vi "Get Column Config.vi"(8 "error in (no error)":errorcluster, 11 "Column Parent in":refnum<class "Column Parent.lvclass">) -> (0 "error out":errorcluster, 2 "Column Configuration":refnum<class "Column Configuration.lvclass">, 3 "Column Parent out":refnum<class "Column Parent.lvclass">)   [LabVIEW 2020, in "Basic Columns.lvlib" / "Column Parent.lvclass"]
uses:
  Column Parent.lvclass
  Column Interface/Column Configuration Interface Class/Column Configuration.lvclass
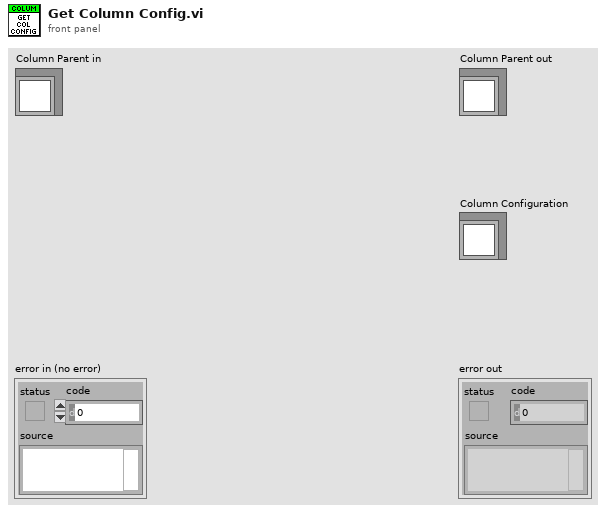
[diagram p1: front panel]
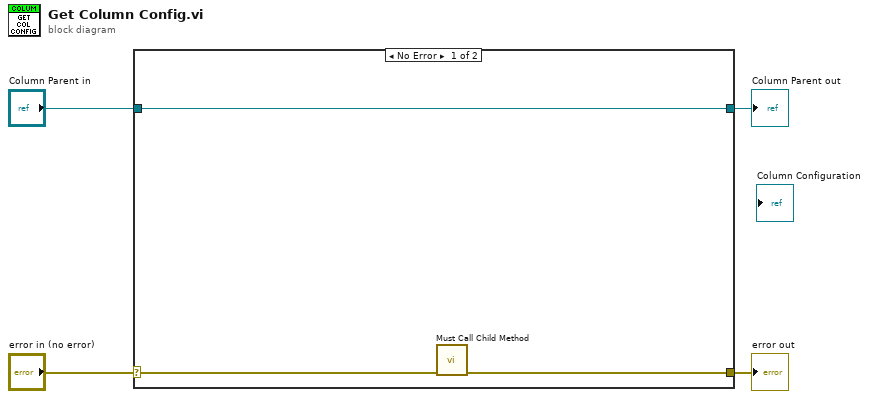
[diagram p0: block diagram]
diagram:
  n1 = case shown="No Error" "error in (no error)" {
    selector: "error in (no error)" -> [w6 w8]
    tunnel: [w7 w9] -> w2
    tunnel: "Column Parent in" -> [w7 w9]
    tunnel: [w5 w8] -> w1
    frame No Error {
      n2 = call "Must Call Child Method.vi"("error in"=w6) -> ("error out"=w5:errorcluster)  [unwired: 10 in]
    }
    frame Error {
    }
  }
  "error out" <- w1
  "Column Parent out" <- w2
